vi "ITX to HDF5.vi"(8 "error in (no error)":errorcluster, 11 "file (use dialog)":path=path "C:/") -> (0 "error out":errorcluster)   [LabVIEW 2016]
uses:
  Data/Data.lvclass
  Data/Typedefs/File Type--enum.ctl
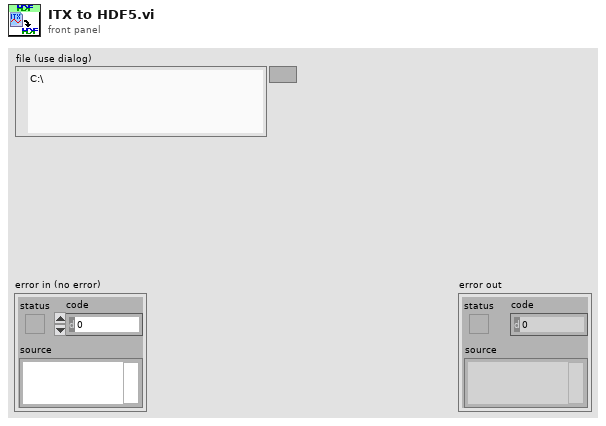
[diagram p1: front panel]
types:
  T1 = typedef "Data.lvclass/File Type--enum.ctl" = enum16{"DAT", "ITX", "HDF5", "TDMS", "VI", "PGSQL"}
  T2 = typedef "Data.lvclass/Dictionary--cluster.ctl" = cluster{"key":string, "value":variant}
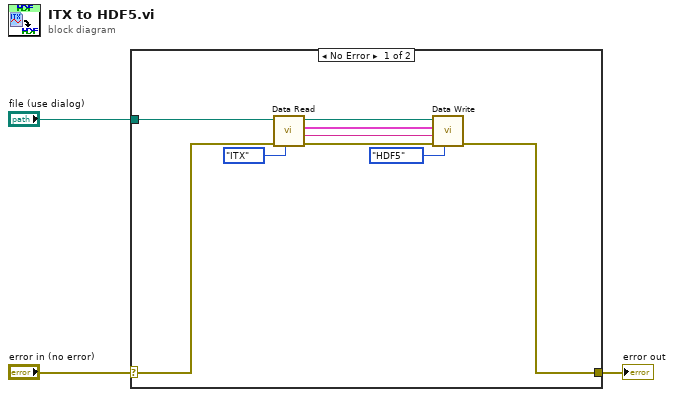
[diagram p0: block diagram]
diagram:
  n1 = case shown="No Error" "error in (no error)" {
    selector: "error in (no error)" -> [w7 w13]
    tunnel: [w6 w13] -> w2
    tunnel: "file (use dialog)" -> [w12 _]
    frame No Error {
      n2 = call "Data Read.vi"("Append Index"=File_Type--enum."ITX" ("File Type"), "error in (no error)"=w7, "path"=w12) -> ("error out"=w10:errorcluster, "Notes"=w9:string, "Data (Dictionary)"=w8:T2[], "path out"=w11:path)  [unwired: 5 in]
      n3 = call "Data Write.vi"("Append Index"=File_Type--enum."HDF5" ("File Type"), "error in (no error)"=w10, "Notes"=w9, "Data (Dictionary)"=w8, "path"=w11) -> ("error out"=w6:errorcluster)  [unwired: 5 in, 1 out]
    }
    frame Error {
    }
  }
  "error out" <- w2
